vi "Autonomous Independent.vi"   [LabVIEW 2019]
doc: "This VI is called when autonomous begins, and will automatically be terminated when autonomous ends. You can carry out timed or sensor driven robot movement independently without needing to return to the caller."
uses:
  <vilib>/Rock Robotics/Network Tables/NT Read String.vi
  Functions/Global Variables/Trajectory Enabled.vi
  <vilib>/Rock Robotics/Network Tables/NT Write Number.vi
  Functions/Global Variables/Robot State.vi
panel:
  # "Be sure to right-click and choose Data Operations>>Make Current Value default if you want to save the array values with the VI"
  # "Edit Select trajecoty to choose what to do here"
types:
  T1 = typedef "Robot State.ctl" = cluster{"Drive System State":T2, "Enable Actions":T5, "Lift System Actions":T6, "SpinnerActions":T7, "Ball System Actions":T8, "Camera Control":bool}
  T2 = typedef "Robot Pivot Motion Commands.ctl" = cluster{"Front Right":T3, "Front Left":T3, "Rear Left":T3, "Rear Right":T3, "Drive Mode":T4, "Reset Drive Encoder":bool}
  T3 = typedef "Pivot Motor Commands.ctl" = cluster{"Drive Power":dbl, "Drive Distance (in)":dbl, "Drive Distance Error (in)":dbl, "Steer Power":dbl, "Steer Angle (deg)":dbl, "Steer Angle Error (deg)":dbl}
  T4 = typedef "Robot Drive Mode.ctl" = enum16{"Velocity", "Distance"}
  T5 = typedef "Enable Actions.ctl" = cluster{"Manual Swerve Drive":bool, "Color System":bool, "Ball System":bool, "Lift System":bool}
  T6 = typedef "Lift System Actions.ctl" = cluster{"Arm Deploy Piston":bool, "Enable Lift Arm":bool, "Enable Climber":bool, "Climber Velocity":dbl, "Lift Arm Velocity":dbl}
  T7 = typedef "Spinner Actions.ctl" = cluster{"Manual Mode ":bool, "Auto rotate n times":bool, "Auto rotate to color\t":bool, "Extend and Retract Arm\t":bool, "Manual Rotation Speed":dbl}
  T8 = typedef "Ball System Actions.ctl" = cluster{"Intake Piston ":bool, "Shoot Ball":bool, "Tube up one Increment\t":bool, "Reverse Ball Intake":bool, "Tube Piston":bool, "Enable Manual Tube":bool, "Tube up four Increments":bool, "Manual Tube Velocity":dbl, "Ball Intake Speed":dbl, "Color Wheel (Shooter)":bool, "Reverse Shooter":bool}
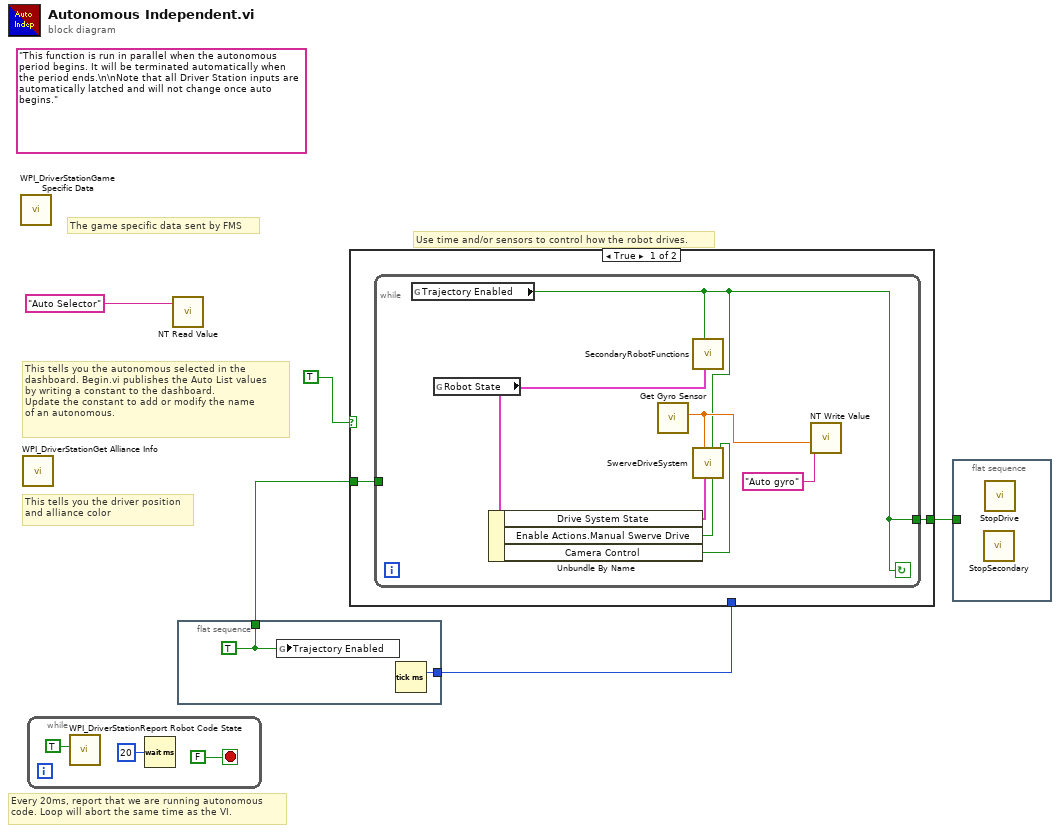
[diagram p0: block diagram]
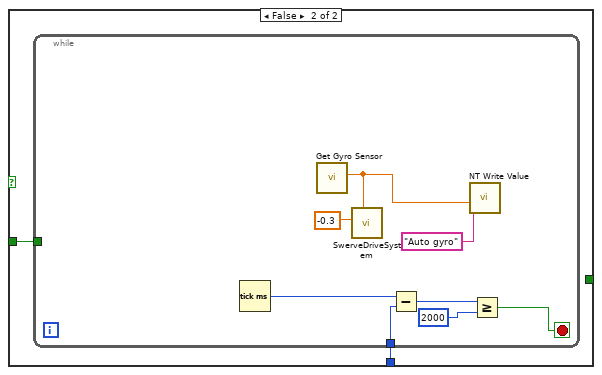
[diagram p2: hidden frame]
diagram:
  (unwired) "This function is run in parallel when the autonomous period begins. It will be terminated automatically when the period ends.\n\nNote that all Driver Station inputs are automatically latched and will not change once auto begins."
  # "The game specific data sent by FMS"
  # "This tells you the autonomous selected in the \ndashboard. Begin.vi publishes the Auto List values\nby writing a constant to the dashboard.\nUpdate the constant to add or modify the name\nof an autonomous."
  # "Every 20ms, report that we are running autonomous\ncode. Loop will abort the same time as the VI."
  # "Use time and/or sensors to control how the robot drives."
  # "This tells you the driver position\nand alliance color"
  n1 = call <vilib>:"WPI_DriverStationGame Specific Data.vi"() -> ()  [unwired: 11 in, 1 out]
  n2 = call <vilib>:"WPI_DriverStationGet Alliance Info.vi"() -> ()  [unwired: 12 out]
  n3 = while {
    stop <- FALSE stop-if-true
    n4 = call <vilib>:"WPI_DriverStationReport Robot Code State.vi"("Autonomous"=TRUE) -> ()  [unwired: 10 in, 1 out]
    n5 = Wait (ms)(milliseconds to wait=u32 20) -> ()  [unwired: 1 out]
  }
  n6 = call-poly <vilib>:"NT Read Value.vi"("Name"="Auto Selector") -> ()  [unwired: 9 in, 2 out]
  n7 = flat-sequence {
    tunnel: [w10] -> w4
    tunnel: [w9] -> w2
    frame #0 {
      w10 = TRUE ("Trajectory Enabled")
      n8 = global write "Trajectory Enabled.vi" "Trajectory Enabled"(w10) -> ()
      n9 = Tick Count (ms)() -> (millisecond timer value=w9:u32)
    }
  }
  n10 = case shown="True" TRUE {
    tunnel: w4 -> [w12 w21]
    tunnel: [w11 _] -> w3
    tunnel: w2 -> [_ w20]
    frame True {
      n11 = while {
        tunnel: w12 -> [_]
        tunnel: [w13] -> w11
        stop <- w13 continue-if-true
        n12 = global read "Trajectory Enabled.vi" "Trajectory Enabled"() -> (w13:bool)
        n13 = global read "Robot State.vi" "Robot State"() -> (w19:T1)
        n14 = Unbundle By Name(w19) -> ("Drive System State"=w18:T2, "Enable Actions.Manual Swerve Drive"=w17:bool, "Camera Control"=w16:bool)
        n15 = call "Get Gyro Sensor.vi"() -> ("Robot Field Orientation (deg)"=w15:dbl)  [unwired: 11 in]
        n16 = call "SecondaryRobotFunctions.vi"("Robot State"=w19, "Automatic State Control Mode (F)"=w13) -> ()  [unwired: 10 in]
        n17 = call "SwerveDriveSystem.vi"("Autonomous Camera Control"=w16, "Enable Auto Swerve Drive"=w17, "Automatic State Control Mode (F)"=w13, "Robot Motion Commands"=w18, "Robot field orientation (deg)"=w15) -> ()  [unwired: 7 in]
        n18 = call-poly <vilib>:"NT Write Value.vi"("Numeric"=w15, "Name"="Auto gyro") -> ()  [unwired: 9 in, 1 out]
      }
    }
    frame False {
      n19 = while {
        tunnel: w21 -> [_]
        tunnel: w20 -> [w25]
        stop <- w22 stop-if-true
        n20 = Tick Count (ms)() -> (millisecond timer value=w26:u32)
        n21 = call "Get Gyro Sensor.vi"() -> ("Robot Field Orientation (deg)"=w29:dbl)  [unwired: 11 in]
        n22 = call "SwerveDriveSystem.vi"("Robot field orientation (deg)"=w29, "Forward"=-0.3) -> ()  [unwired: 10 in]
        n23 = Subtract(x=w26, y=w25) -> (x-y=w24:u32)
        n24 = call-poly <vilib>:"NT Write Value.vi"("Numeric"=w29, "Name"="Auto gyro") -> ()  [unwired: 9 in, 1 out]
        n25 = Greater Or Equal?(x=w24, y=u32 2000) -> (x >= y?=w22:bool)
      }
    }
  }
  n26 = flat-sequence {
    tunnel: w3 -> [_]
    frame #0 {
      n27 = call "StopSecondary.vi"() -> ()  [unwired: 12 in]
      n28 = call "StopDrive.vi"() -> ()  [unwired: 3 in]
    }
  }
